vi "video.vi"() -> ()   [LabVIEW 2017]
uses:
  <vilib>/userdefined/High Color/IMAQdx.ctl
  <vilib>/myRIO/Instrument Drivers/Onboard IO/PWM/typedefs/PWM Reference.ctl
  <vilib>/myRIO/Common/Instrument Driver Framework/Utilities/typedefs/myRIO Generic Hardware Reference.ctl
  <vilib>/myRIO/Common/Instrument Driver Framework/Utilities/typedefs/Hardware Version Enum.ctl
  <vilib>/myRIO/Common/Instrument Driver Framework/Utilities/typedefs/myRIO v1.0 Reference.ctl
  <vilib>/myRIO/Common/Instrument Driver Framework/Utilities/typedefs/Generic FPGA Reference.ctl
  <vilib>/myRIO/Common/Instrument Driver Framework/myRIO v1.0/PWM/typedefs/PWM Channels Enum.ctl
  <vilib>/myRIO/Instrument Drivers/Onboard IO/PWM/typedefs/PWM Configuration.ctl
  <vilib>/userdefined/High Color/nirio_resource_hc.ctl
  <vilib>/myRIO/Common/Instrument Driver Framework/Utilities/vis/Is FPGA Ref Available.vi
  <vilib>/myRIO/Common/Instrument Driver Framework/myRIO v1.0/PWM/vis/myRIO v1.1 Open PWM.vi
  <vilib>/myRIO/Instrument Drivers/Onboard IO/PWM/vis/Set Duty Cycle and Frequency.vi
  <vilib>/myRIO/Common/Instrument Driver Framework/Utilities/vis/Validate Channels.vi
  <vilib>/myRIO/Common/Instrument Driver Framework/myRIO v1.0/PWM/vis/myRIO v1.0 Reserve PWM.vi
  <vilib>/myRIO/Common/Instrument Driver Framework/myRIO v1.0/UART/vis/myRIO v1.0 Close UART.vi
  <vilib>/myRIO/Common/Instrument Driver Framework/myRIO v1.0/PWM/vis/myRIO v1.0 Build MUX Configuration PWM.vi
  <vilib>/myRIO/Common/Instrument Driver Framework/myRIO v1.0/Resource Manager/vis/myRIO v1.0 Reserve Channel List.vi
  <vilib>/myRIO/Common/Instrument Driver Framework/myRIO v1.0/Resource Manager/vis/myRIO v1.0 Create Configuration List.vi
  <vilib>/myRIO/Common/Instrument Driver Framework/myRIO v1.0/Resource Manager/vis/myRIO v1.0 Reserve Channel.vi
  <vilib>/myRIO/Common/Instrument Driver Framework/myRIO v1.0/Resource Manager/vis/myRIO v1.0 Unreserve Channel.vi
  <vilib>/myRIO/Common/Instrument Driver Framework/myRIO v1.0/Resource Manager/vis/myRIO v1.0 Build Mutex Name.vi
  <vilib>/Utility/VariantDataType/GetNumericInfo.vi
  <vilib>/Utility/error.llb/Error Cluster From Error Code.vi
  <vilib>/myRIO/Common/Instrument Driver Framework/myRIO v1.0/myRIO v1.1 Open.vi
  <vilib>/myRIO/Common/Instrument Driver Framework/Utilities/vis/IO Manager.vi
  <vilib>/myRIO/Common/Instrument Driver Framework/Utilities/vis/Configuration Manager.vi
  <vilib>/myRIO/Common/Instrument Driver Framework/myRIO v1.0/Resource Manager/vis/myRIO v1.0 Configure IO.vi
  <vilib>/myRIO/Common/Instrument Driver Framework/myRIO v1.0/myRIO v1.0 Close.vi
  <vilib>/myRIO/Common/Instrument Driver Framework/myRIO v1.0/PWM/vis/myRIO v1.0 Write PWM.vi
  <vilib>/myRIO/Common/Instrument Driver Framework/Utilities/vis/FPGA Ref Manager.vi
  <vilib>/myRIO/Common/Instrument Driver Framework/myRIO v1.0/myRIO v1.0 Reset FPGA.vi
  <vilib>/myRIO/Common/Instrument Driver Framework/myRIO v1.0/IRQ/vis/myRIO v1.0 IRQ Info FGV.vi
  <vilib>/myRIO/Common/Instrument Driver Framework/myRIO v1.0/IRQ/vis/myRIO v1.0 Timer IRQ Info FGV.vi
  <vilib>/myRIO/Common/Instrument Driver Framework/myRIO v1.0/IRQ/vis/myRIO v1.0 ISR Agent.vi
  <vilib>/myRIO/Express VI/Onboard IO/PWM/PWM Express VI.xnode
  <vilib>/myRIO/Instrument Drivers/Onboard IO/PWM/vis/myRIO PWM Open.xnode
  <vilib>/vision/driver/NI_Vision_Acquisition_Software.lvlib
  <vilib>/myRIO/Instrument Drivers/Onboard IO/PWM/PWM.lvlib
  <vilib>/myRIO/Instrument Drivers/Utilities/Utilities.lvlib
panel:
  out "pass":sgl
  in  "stop":bool
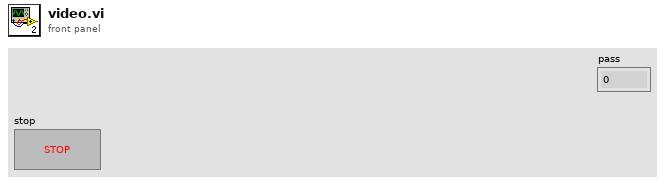
[diagram p1: front panel]
types:
  T1 = typedef "IMAQdx.ctl" = refnum<k21>
  T2 = typedef "IMAQ Image.ctl" = refnum<image>
  T3 = typedef "PWM.lvlib/PWM Reference.ctl" = cluster{"myRIO Reference":T4, "PWM Channels Enum":T8, "PWM Configuration":T9}
  T4 = typedef "myRIO Generic Hardware Reference.ctl" = cluster{"myRIO Model":T5, "myRIO Hardware Reference":T6}
  T5 = typedef "Hardware Version Enum.ctl" = enum16{"Unknown", "myRIO-1900", "myRIO-1950", "roboRIO", "NI ELVIS RIO CM"}
  T6 = typedef "myRIO v1.0 Reference.ctl" = cluster{"Generic FPGA Reference":T7, "Allow multiple opens":bool}
  T7 = typedef "Generic FPGA Reference.ctl" = refnum<k20>
  T8 = typedef "PWM Channels Enum.ctl" = enum16{"Not Connected", "C/PWM0", "C/PWM1", "A/PWM0", "A/PWM1", "A/PWM2", "B/PWM0", "B/PWM1", "B/PWM2", "PWM/PWM0", "PWM/PWM1", "PWM/PWM2", "PWM/PWM3", "PWM/PWM4", "PWM/PWM5", "PWM/PWM6", "PWM/PWM7", "PWM/PWM8", "PWM/PWM9"}
  T9 = typedef "PWM.lvlib/PWM Configuration.ctl" = cluster{"Frequency":dbl, "Duty Cycle":dbl}
  T10 = typedef "nirio_resource_hc.ctl" = tag
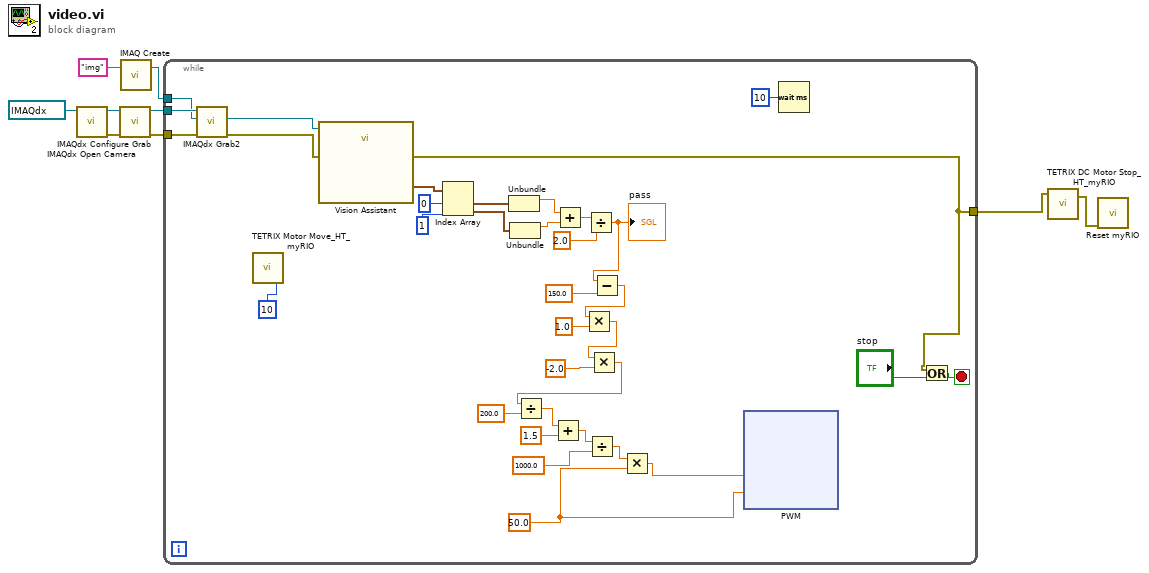
[diagram p0: block diagram]
diagram:
  n1 = call <vilib>:"IMAQdx Open Camera.vi"("Session In"=T1 "cam0") -> ("error out"=w4:errorcluster, "Session Out"=w8:T1)  [unwired: 9 in]
  n2 = call <vilib>:"IMAQdx Configure Grab.vi"("error in"=w4, "Session In"=w8) -> ("error out"=w3:errorcluster, "Session Out"=w7:T1)  [unwired: 8 in]
  n3 = call "IMAQ Create"("Image Name"="img") -> ("New Image"=w5:T2)  [unwired: 4 in, 1 out]
  n4 = while {
    tunnel: w7 -> [w43]
    tunnel: w5 -> [w42]
    tunnel: w3 -> [w41]
    tunnel: [w23] -> w1
    stop <- w37 stop-if-true
    w15 = sgl 50.0 ("y")
    n5 = call <vilib>:"IMAQdx Grab2.vi"("error in"=w41, "Image In"=w42, "Session In"=w43) -> ("error out"=w39:errorcluster, "Image Out"=w40:T2)  [unwired: 5 in, 2 out]
    n6 = call <vilib>:"TETRIX Motor Move_HT_myRIO.vi"("Power (-100 to 100)\n0 = Stop/Brake\n-128 = Stop/Coast"=i8 10 ("Power (-100 to 100)\n0 = Stop/Brake\n-128 = Stop/Coast")) -> ()  [unwired: 6 in, 1 out]
    n7 = call "Vision Assistant"("Image In"=w40, "error in"=w39) -> ("Edges Coordinates (Edge Detector 1)"=w36:cluster{"X":sgl, "Y":sgl}[], "error out"=w23:errorcluster)  [unwired: 23 in, 1 out]
    n8 = Index Array(array=w36, index #1=0 ("index"), index #2=1 ("index")) -> (element #1=w33:cluster{"X":sgl, "Y":sgl}, element #2=w32:cluster{"X":sgl, "Y":sgl})
    n9 = Unbundle(w33) -> ("X"=w30:sgl)  [unwired: 1 out]
    n10 = Unbundle(w32) -> ("X"=w31:sgl)  [unwired: 1 out]
    n11 = Add(x=w30, y=w31) -> (x+y=w29:sgl)
    n12 = Divide(x=w29, y=sgl 2.0) -> (x/y=w21:sgl)
    "pass" <- w21
    n13 = Subtract(x=w21, y=sgl 150.0) -> (x-y=w12:sgl)
    n14 = Multiply(x=w12, y=sgl 1.0) -> (x*y=w13:sgl)
    n15 = Multiply(x=w13, y=sgl -2.0) -> (x*y=w20:sgl)
    n16 = Divide(x=w20, y=sgl 200.0) -> (x/y=w26:sgl)
    n17 = Add(x=w26, y=sgl 1.5) -> (x+y=w25:sgl)
    n18 = Divide(x=w25, y=sgl 1000.0) -> (x/y=w24:sgl)
    n19 = Multiply(x=w24, y=w15) -> (x*y=w27:sgl)
    n20 = xnode "PWM"("Duty Cycle"=w27, "Frequency [Hz]"=w15) -> ()  [unwired: 1 in, 1 out]
    n21 = Wait (ms)(milliseconds to wait=u32 10) -> ()  [unwired: 1 out]
    n22 = Or(x=w23, y="stop") -> (x .or. y?=w37:bool)
  }
  n23 = call <vilib>:"TETRIX DC Motor Stop_HT_myRIO.vi"("error in (no error)"=w1) -> ("error out"=w2:errorcluster)  [unwired: 3 in]
  n24 = call <vilib>:"Reset myRIO.vi"("error in (no error)"=w2) -> ()  [unwired: 10 in, 1 out]
